vi "INI_Read Data LabVIEW ini File.vi"(8 "Error":errorcluster) -> (0 "Error Out":errorcluster={"status"=TRUE, "code"=1055, "source"="Property Node in Windows.vi->Populate Font ComboBox.vi->Populate Font Control.vi->ReadDataFromLabVIEWINI.vi"}, 3 "INI Data Out":T1={"Show Layer Tab?"=FALSE, "Show Terminals?"=FALSE, "Text"={"Font"="Small Fonts", "Alignment"=0, "Size"=9}, "3rd party Templates"={"Store 3rd party Templates?"=TRUE, "Folder Name"="3rd party"}, "Merge user layers on commit"=TRUE, "Body Text"={"Line 1 text"="", "Line 2 text"="", "Line 3 text"="", "Line 4 text"="", "Line 1 color"=0, "Line 2 color"=0, "Line 3 color"=0, "Line 4 color"=0, "Body Text Spec"={"Font"="", "Alignment"=0, "Size"=3}, "Center text vertically"=FALSE, "Capitalize Text"=FALSE}, "Fill Color"=16711680, "Edge Color"=0, "Tab"=0, "Tool"=enum."Ellipse", "Disable Layers?"=FALSE} {"Body Text"."Body Text Spec"."Alignment" items=["left", "center", "right"]; "Text"."Alignment" items=["left", "center", "right"]})   [LabVIEW 2021]
uses:
  TypeDefs/Cluster_INI Data.ctl
  vi.lib/LabVIEW Icon API/lv_icon/Controls/Font.ctl
  vi.lib/LabVIEW Icon API/lv_icon/Controls/Alignment.ctl
  TypeDefs/Num_Font Size.ctl
  TypeDefs/Cluster_BodyText.ctl
  vi.lib/LabVIEW Icon API/lv_icon/Controls/IEColor.ctl
  TypeDefs/Cluster_Button Draw Tools.ctl
  TypeDefs/Bool_Draw Tool.ctl
  TypeDefs/Bool_Line Tool.ctl
  TypeDefs/Bool_ColorExtractor Tool.ctl
  TypeDefs/Bool_Fill Tool.ctl
  TypeDefs/Bool_IERect Tool.ctl
  TypeDefs/Bool_FRect Tool.ctl
  TypeDefs/Bool_Circle Tool.ctl
  TypeDefs/Bool_FillCircle Tool.ctl
  TypeDefs/Bool_Eraser Tool.ctl
  TypeDefs/Bool_Text Tool.ctl
  TypeDefs/Bool_Selection Tool.ctl
  TypeDefs/Bool_Move Tool.ctl
  <resource>/dialog/lvconfig.llb/LV Config Read String.vi
  <resource>/dialog/lvconfig.llb/LV Config Read Color.vi
  <resource>/dialog/lvconfig.llb/LV Config Read Boolean.vi
panel:
  in  "INI Data":T1={"Show Layer Tab?"=TRUE, "Show Terminals?"=FALSE, "Text"={"Font"="Small Fonts", "Alignment"=1, "Size"=9}, "3rd party Templates"={"Store 3rd party Templates?"=TRUE, "Folder Name"="3rd party"}, "Merge user layers on commit"=FALSE, "Body Text"={"Line 1 text"="", "Line 2 text"="", "Line 3 text"="", "Line 4 text"="", "Line 1 color"=0, "Line 2 color"=0, "Line 3 color"=0, "Line 4 color"=0, "Body Text Spec"={"Font"="Small Fonts", "Alignment"=1, "Size"=9}, "Center text vertically"=TRUE, "Capitalize Text"=TRUE}, "Fill Color"=16711680, "Edge Color"=0, "Tab"=0, "Tool"=enum."Pencil", "Disable Layers?"=FALSE} {"Body Text"."Body Text Spec"."Alignment" items=["left", "center", "right"]; "Text"."Alignment" items=["left", "center", "right"]}
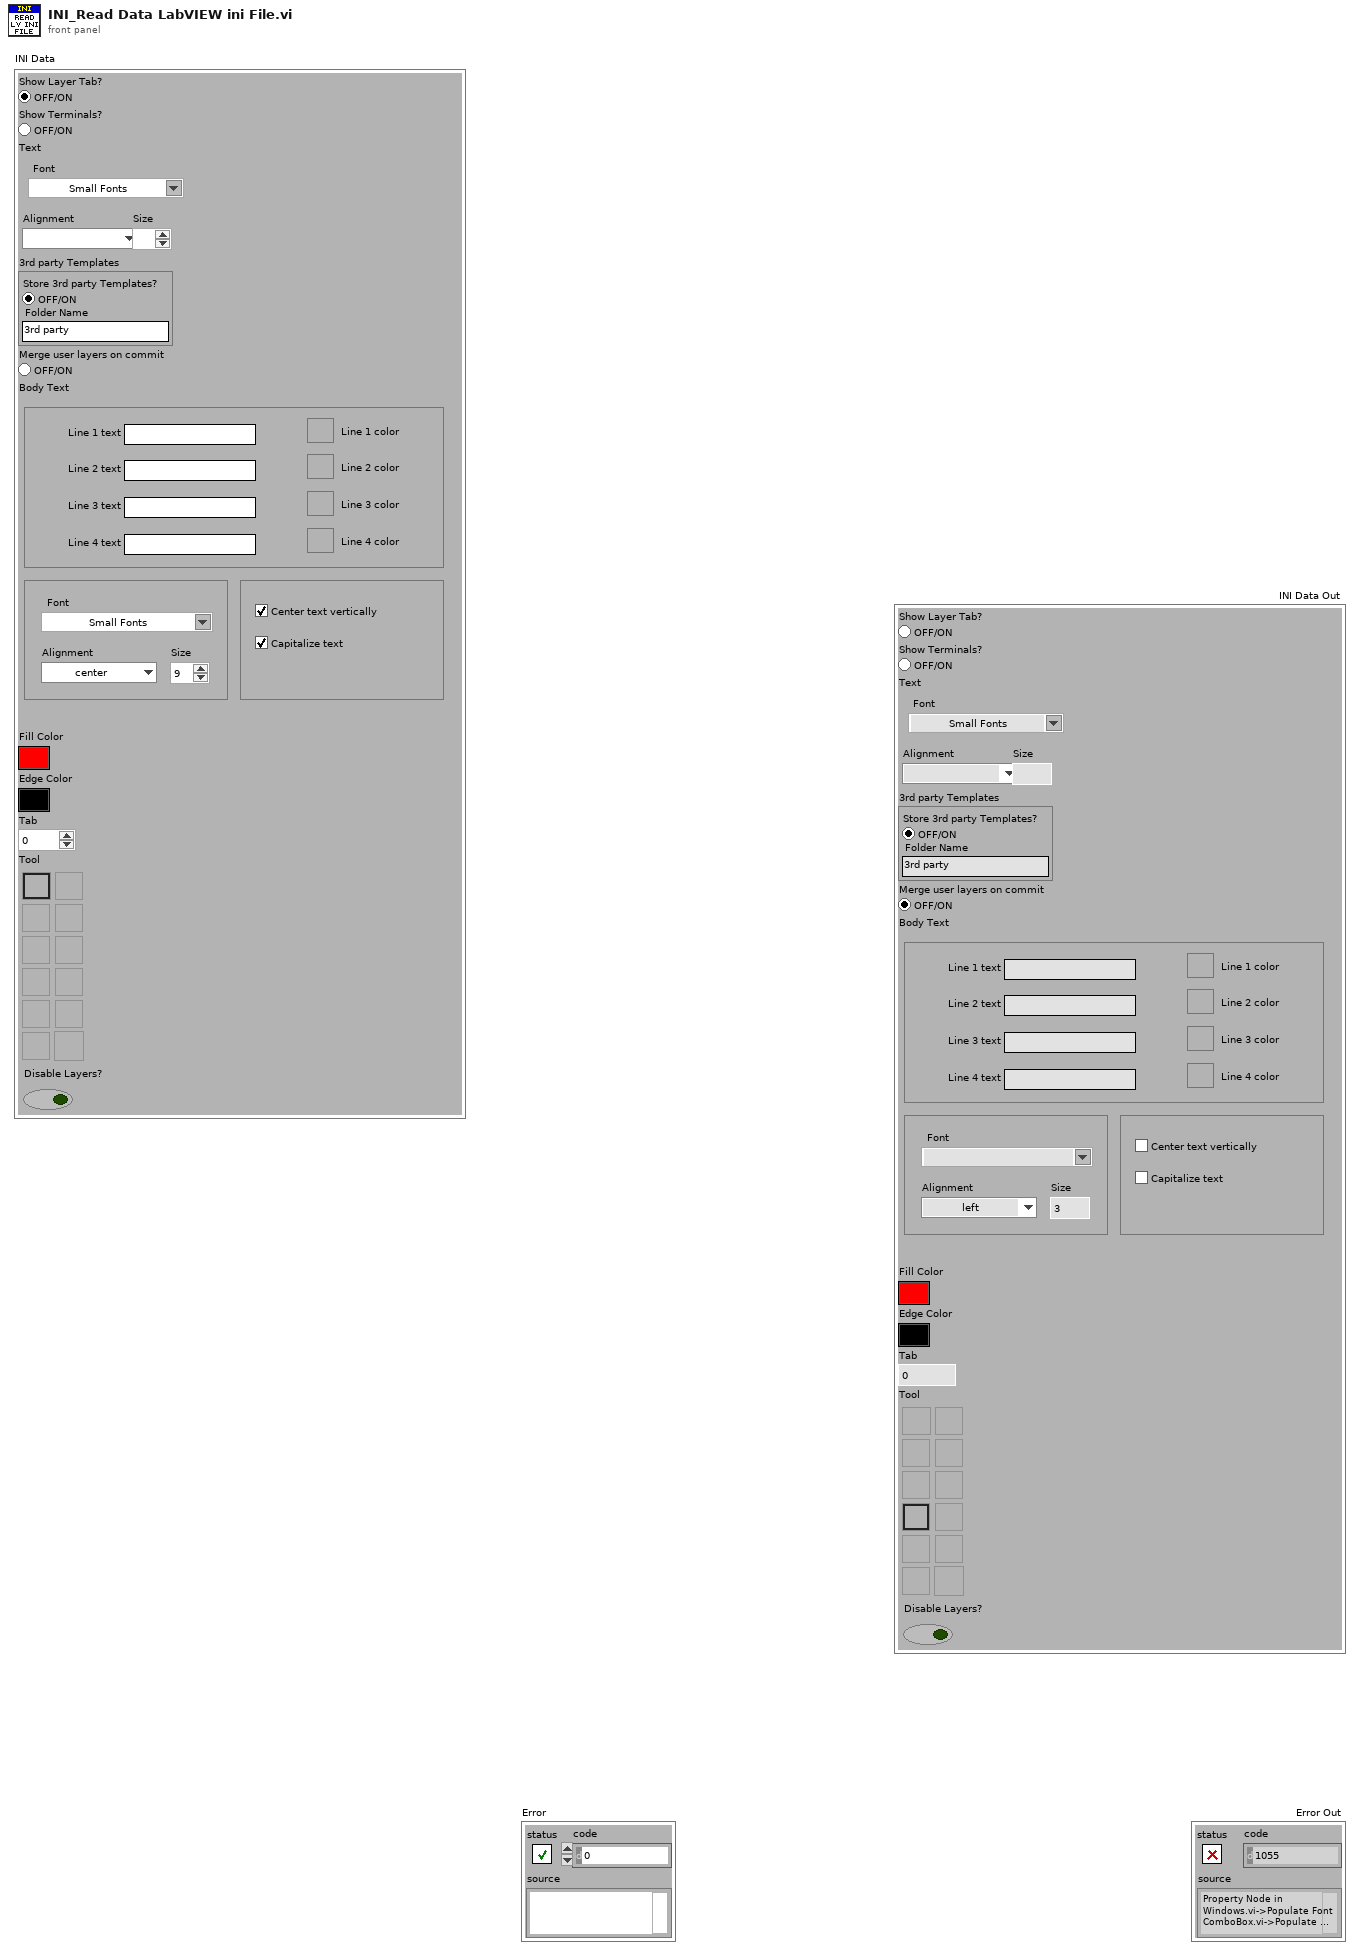
[diagram p1: front panel]
types:
  T1 = typedef "Cluster_INI Data.ctl" = cluster{"Show Layer Tab?":bool, "Show Terminals?":bool, "Text":cluster{"Font":T2, "Alignment":T3, "Size":T4}, "3rd party Templates":cluster{"Store 3rd party Templates?":bool, "Folder Name":string}, "Merge user layers on commit":bool, "Body Text":T5, "Fill Color":T6, "Edge Color":T6, "Tab":u16, "Tool":T7, "Disable Layers?":bool}
  T2 = typedef "Font.ctl" = string
  T3 = typedef "Alignment.ctl" = u16
  T4 = typedef "Num_Font Size.ctl" = u8
  T5 = typedef "Cluster_BodyText.ctl" = cluster{"Line 1 text":string, "Line 2 text":string, "Line 3 text":string, "Line 4 text":string, "Line 1 color":u32, "Line 2 color":u32, "Line 3 color":u32, "Line 4 color":u32, "Body Text Spec":cluster{"Font":T2, "Alignment":T3, "Size":u8}, "Center text vertically":bool, "Capitalize Text":bool}
  T6 = typedef "IEColor.ctl" = u32
  T7 = typedef "Cluster_Button Draw Tools.ctl" = enum32{"Pencil", "Line", "Dropper", "Fill", "Rectangle", "Filled Rectangle", "Ellipse", "Filled Ellipse", "Eraser", "Text", "Select", "Move"}
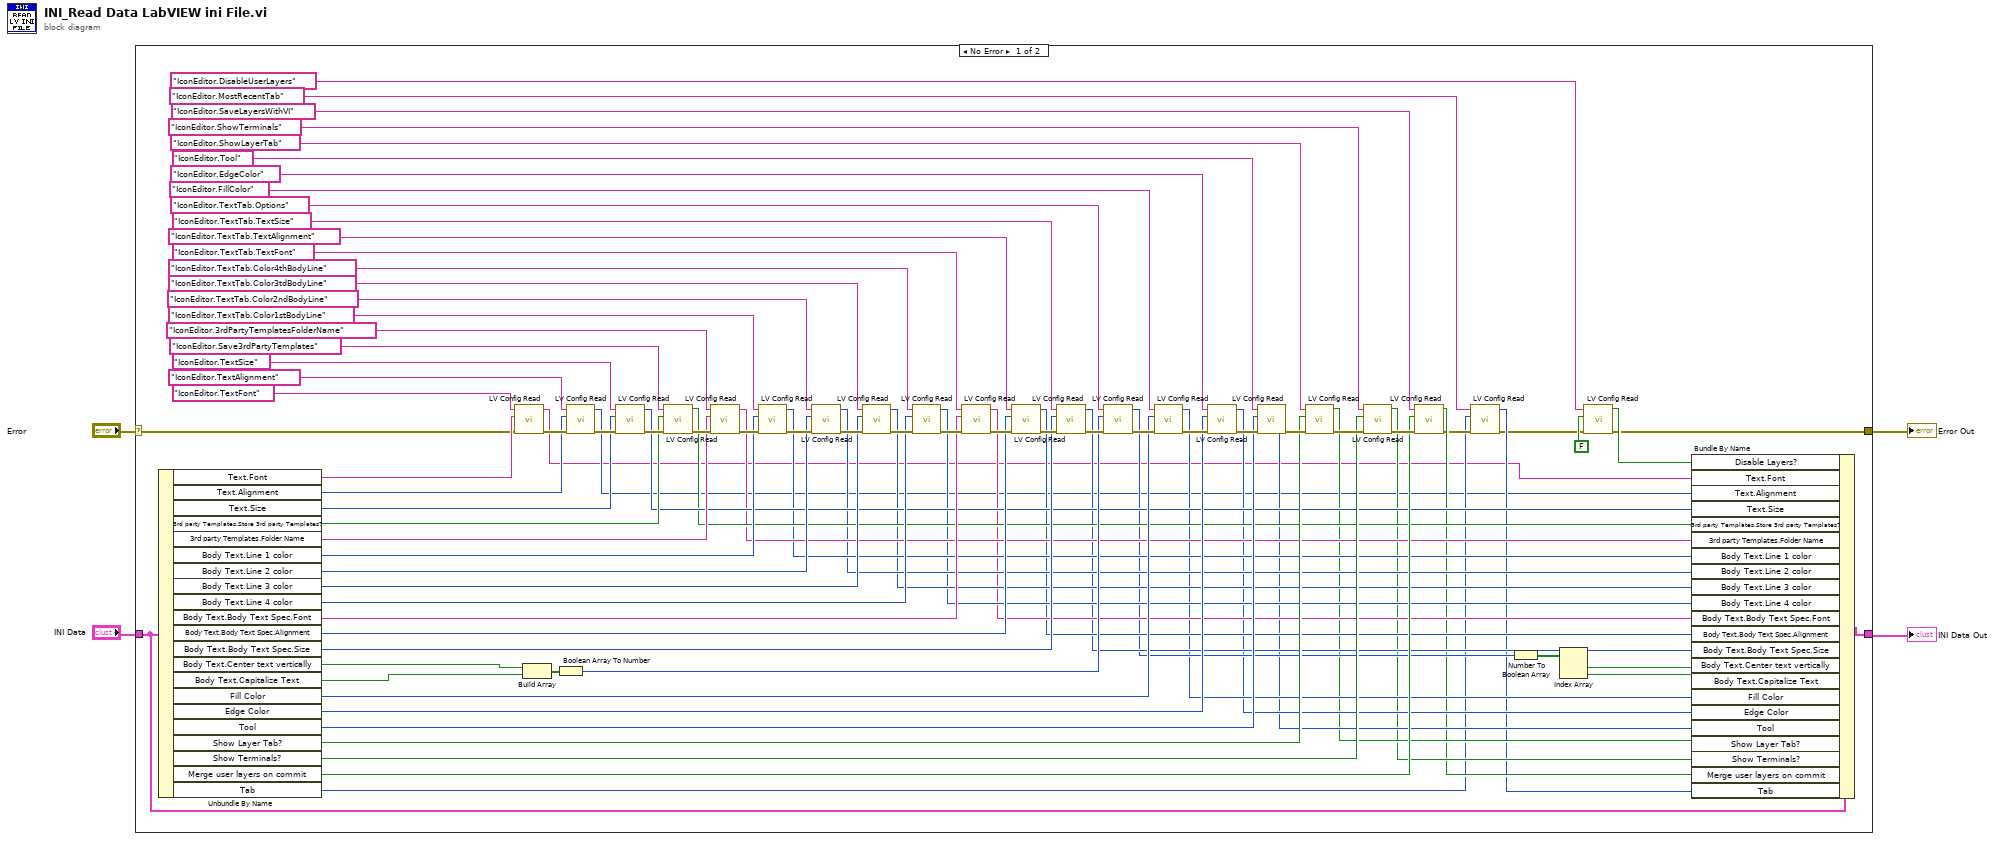
[diagram p0: block diagram]
diagram:
  n1 = case shown="No Error" "Error" {
    selector: "Error" -> [w14 w98]
    tunnel: [w5 w98] -> w3
    tunnel: "INI Data" -> [w19 _]
    tunnel: [w20 _] -> w2
    frame No Error {
      n2 = Unbundle By Name(w19) -> ("Text.Font"=w60:T2, "Text.Alignment"=w59:T3, "Text.Size"=w58:T4, "3rd party Templates.Store 3rd party Templates?"=w57:bool, "3rd party Templates.Folder Name"=w53:string, "Body Text.Line 1 color"=w52:u32, "Body Text.Line 2 color"=w51:u32, "Body Text.Line 3 color"=w50:u32, "Body Text.Line 4 color"=w49:u32, "Body Text.Body Text Spec.Font"=w48:T2, "Body Text.Body Text Spec.Alignment"=w47:T3, "Body Text.Body Text Spec.Size"=w46:u8, "Body Text.Center text vertically"=w54:bool, "Body Text.Capitalize Text"=w55:bool, "Fill Color"=w44:T6, "Edge Color"=w43:T6, "Tool"=w42:T7, "Show Layer Tab?"=w41:bool, "Show Terminals?"=w40:bool, "Merge user layers on commit"=w39:bool, "Tab"=w16:u16)
      n3 = call-poly <resource>:"LV Config Read.vi"("error in"=w14, "default value"=w60, "key"="IconEditor.TextFont") -> ("error out"=w97:errorcluster, "value"=w7:string)  [unwired: 3 out]
      n4 = Build Array(w54, w55) -> (w56:bool[])
      n5 = Boolean Array To Number(Boolean array=w56) -> (number=w45:u32)
      n6 = call-poly <resource>:"LV Config Read.vi"("error in"=w97, "default value"=w59, "key"="IconEditor.TextAlignment") -> ("error out"=w96:errorcluster, "value"=w11:u32)  [unwired: 3 out]
      n7 = call-poly <resource>:"LV Config Read.vi"("error in"=w96, "default value"=w58, "key"="IconEditor.TextSize") -> ("error out"=w95:errorcluster, "value"=w38:u32)  [unwired: 3 out]
      n8 = call-poly <resource>:"LV Config Read.vi"("error in"=w95, "default value"=w57, "key"="IconEditor.Save3rdPartyTemplates") -> ("error out"=w94:errorcluster, "value"=w37:bool)  [unwired: 3 out]
      n9 = call-poly <resource>:"LV Config Read.vi"("error in"=w94, "default value"=w53, "key"="IconEditor.3rdPartyTemplatesFolderName") -> ("error out"=w93:errorcluster, "value"=w36:string)  [unwired: 3 out]
      n10 = call-poly <resource>:"LV Config Read.vi"("error in"=w93, "default value"=w52, "key"="IconEditor.TextTab.Color1stBodyLine") -> ("error out"=w92:errorcluster, "value"=w35:u32)  [unwired: 3 out]
      n11 = call-poly <resource>:"LV Config Read.vi"("error in"=w92, "default value"=w51, "key"="IconEditor.TextTab.Color2ndBodyLine") -> ("error out"=w91:errorcluster, "value"=w34:u32)  [unwired: 3 out]
      n12 = call-poly <resource>:"LV Config Read.vi"("error in"=w91, "default value"=w50, "key"="IconEditor.TextTab.Color3tdBodyLine") -> ("error out"=w90:errorcluster, "value"=w33:u32)  [unwired: 3 out]
      n13 = call-poly <resource>:"LV Config Read.vi"("error in"=w90, "default value"=w49, "key"="IconEditor.TextTab.Color4thBodyLine") -> ("error out"=w89:errorcluster, "value"=w32:u32)  [unwired: 3 out]
      n14 = call-poly <resource>:"LV Config Read.vi"("error in"=w89, "default value"=w48, "key"="IconEditor.TextTab.TextFont") -> ("error out"=w88:errorcluster, "value"=w31:string)  [unwired: 3 out]
      n15 = call-poly <resource>:"LV Config Read.vi"("error in"=w88, "default value"=w47, "key"="IconEditor.TextTab.TextAlignment") -> ("error out"=w87:errorcluster, "value"=w30:u32)  [unwired: 3 out]
      n16 = call-poly <resource>:"LV Config Read.vi"("error in"=w87, "default value"=w46, "key"="IconEditor.TextTab.TextSize") -> ("error out"=w86:errorcluster, "value"=w29:u32)  [unwired: 3 out]
      n17 = call-poly <resource>:"LV Config Read.vi"("error in"=w86, "default value"=w45, "key"="IconEditor.TextTab.Options") -> ("error out"=w85:errorcluster, "value"=w28:u32)  [unwired: 3 out]
      n18 = call-poly <resource>:"LV Config Read.vi"("error in"=w85, "default value"=w44, "key"="IconEditor.FillColor") -> ("error out"=w84:errorcluster, "value"=w26:u32)  [unwired: 3 out]
      n19 = call-poly <resource>:"LV Config Read.vi"("error in"=w84, "default value"=w43, "key"="IconEditor.EdgeColor") -> ("error out"=w83:errorcluster, "value"=w25:u32)  [unwired: 3 out]
      n20 = call-poly <resource>:"LV Config Read.vi"("error in"=w83, "default value"=w42, "key"="IconEditor.Tool") -> ("error out"=w82:errorcluster, "value"=w24:u32)  [unwired: 3 out]
      n21 = call-poly <resource>:"LV Config Read.vi"("error in"=w82, "default value"=w41, "key"="IconEditor.ShowLayerTab") -> ("error out"=w81:errorcluster, "value"=w23:bool)  [unwired: 3 out]
      n22 = call-poly <resource>:"LV Config Read.vi"("error in"=w81, "default value"=w40, "key"="IconEditor.ShowTerminals") -> ("error out"=w62:errorcluster, "value"=w22:bool)  [unwired: 3 out]
      n23 = call-poly <resource>:"LV Config Read.vi"("error in"=w62, "default value"=w39, "key"="IconEditor.SaveLayersWithVI") -> ("error out"=w18:errorcluster, "value"=w21:bool)  [unwired: 3 out]
      n24 = call-poly <resource>:"LV Config Read.vi"("error in"=w18, "default value"=w16, "key"="IconEditor.MostRecentTab") -> ("error out"=w6:errorcluster, "value"=w15:u32)  [unwired: 3 out]
      n25 = Number To Boolean Array(number=w28) -> (Boolean array=w27:bool[])
      n26 = Index Array(array=w27) -> (element #1=w13:bool, element #2=w12:bool)  [unwired: 2 in]
      n27 = call-poly <resource>:"LV Config Read.vi"("error in"=w6, "default value"=FALSE ("value"), "key"="IconEditor.DisableUserLayers") -> ("error out"=w5:errorcluster, "value"=w9:bool)  [unwired: 1 in, 2 out]
      n28 = Bundle By Name(cluster=w19, "Disable Layers?"=w9, "Text.Font"=w7, "Text.Alignment"=w11, "Text.Size"=w38, "3rd party Templates.Store 3rd party Templates?"=w37, "3rd party Templates.Folder Name"=w36, "Body Text.Line 1 color"=w35, "Body Text.Line 2 color"=w34, "Body Text.Line 3 color"=w33, "Body Text.Line 4 color"=w32, "Body Text.Body Text Spec.Font"=w31, "Body Text.Body Text Spec.Alignment"=w30, "Body Text.Body Text Spec.Size"=w29, "Body Text.Center text vertically"=w13, "Body Text.Capitalize Text"=w12, "Fill Color"=w26, "Edge Color"=w25, "Tool"=w24, "Show Layer Tab?"=w23, "Show Terminals?"=w22, "Merge user layers on commit"=w21, "Tab"=w15) -> (w20:T1)
    }
    frame Error {
    }
  }
  "Error Out" <- w3
  "INI Data Out" <- w2
